vi "DG645_control.vi"() -> ()   [LabVIEW 2016]
uses:
  <vilib>/Utility/xml.llb/Write to XML File(string).vi
  <vilib>/Utility/xml.llb/Read From XML File(string).vi
  <instrlib>/Stanford Research DG645/Stanford Research DG645.lvlib
panel:
  in  "Singl shot":bool
  out "Digital Waveform Graph":digitalwaveform(graph)={"t0"=timestamp(0 s since 1904-01-01), "dt"=4.817138671875e-08, "Y"={"transitions"=[], "data"=array4096x5[20480 elements]}}
  out "Updating":bool
  out "Error":bool
  in  "Reset on update?":bool
  in  "Stop":bool
  in  "Trigger Source":u16(ring)=6 items=["Internal", "External rising edge", "External falling edge", "Single shot internal rising edge", "Single shot external rising edge", "Single shot", "Line"]
  in  "Export to File":bool
  in  "Import From File":bool
  in  "Update Device":bool
  out "error out":errorcluster
  in  "Delays":T1(array[cluster])=[{"Channel"=2, "Reference"=0, "Delay Time"=1e-08}, {"Channel"=3, "Reference"=2, "Delay Time"=1e-05}, {"Channel"=4, "Reference"=2, "Delay Time"=0.000186}, {"Channel"=5, "Reference"=4, "Delay Time"=1e-05}, {"Channel"=6, "Reference"=4, "Delay Time"=3e-07}, {"Channel"=7, "Reference"=6, "Delay Time"=1e-05}, {"Channel"=8, "Reference"=6, "Delay Time"=1e-06}, {"Channel"=9, "Reference"=8, "Delay Time"=1e-05}] {"Delay Time" format="%#_6p"; "Reference" items=["T0"=0, "A"=2, "B"=3, "C"=4, "D"=5, "E"=6, "F"=7, "G"=8, "H"=9]; "Channel" items=["A"=2, "B"=3, "C"=4, "D"=5, "E"=6, "F"=7, "G"=8, "H"=9]}
  in  "Trigger Rate":dbl=50.0
  in  "Outputs":T2(array[cluster])=[{"Output"=0, "Offset"=0.0, "Level"=5.0, "Polarity"=TRUE, "Prescale Factor"=2, "Prescale Phase"=0, "Description"="valve"}, {"Output"=1, "Offset"=0.0, "Level"=5.0, "Polarity"=TRUE, "Prescale Factor"=1, "Prescale Phase"=0, "Description"="flash lamp"}, {"Output"=2, "Offset"=0.0, "Level"=2.7, "Polarity"=TRUE, "Prescale Factor"=1, "Prescale Phase"=0, "Description"="q-switch"}, {"Output"=3, "Offset"=0.0, "Level"=5.0, "Polarity"=TRUE, "Prescale Factor"=1, "Prescale Phase"=0, "Description"="ramp"}, {"Output"=4, "Offset"=0.0, "Level"=5.0, "Polarity"=TRUE, "Prescale Factor"=1, "Prescale Phase"=0, "Description"="scope"}] {"Output" items=["T0", "Output AB", "Output CD", "Output EF", "Output GH"]; "Offset" format="%#_13g"; "Prescale Phase" max=1073741822; "Prescale Factor" min=1 max=1073741823}
  in  "VISA resource name":refnum<visa-resource-name>="DG645_HOGAN"
  # "DG645 control"
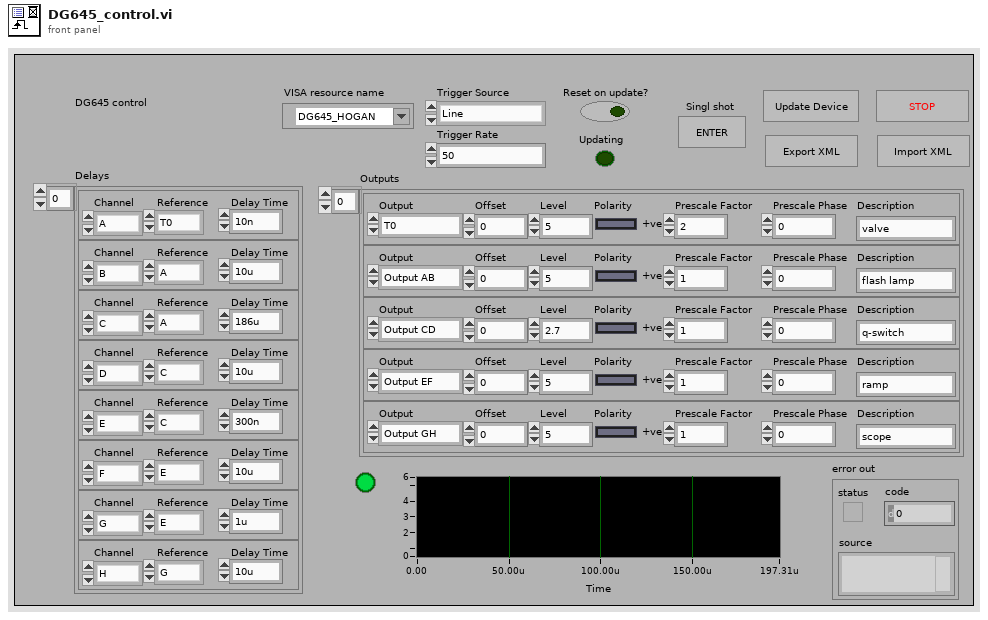
[diagram p1: front panel]
types:
  T1 = cluster{"Channel":u16, "Reference":u16, "Delay Time":dbl}[]
  T2 = cluster{"Output":u16, "Offset":dbl, "Level":dbl, "Polarity":bool, "Prescale Factor":u32, "Prescale Phase":u32, "Description":string}[]
  T3 = cluster{"VISA resource name":refnum<visa-resource-name>, "Trigger Source":u16, "Trigger Rate":dbl, "Delays":cluster{"Channel":u16, "Reference":u16, "Delay Time":dbl}[], "Outputs":cluster{"Output":u16, "Offset":dbl, "Level":dbl, "Polarity":bool, "Prescale Factor":u32, "Prescale Phase":u32, "Description":string}[]}
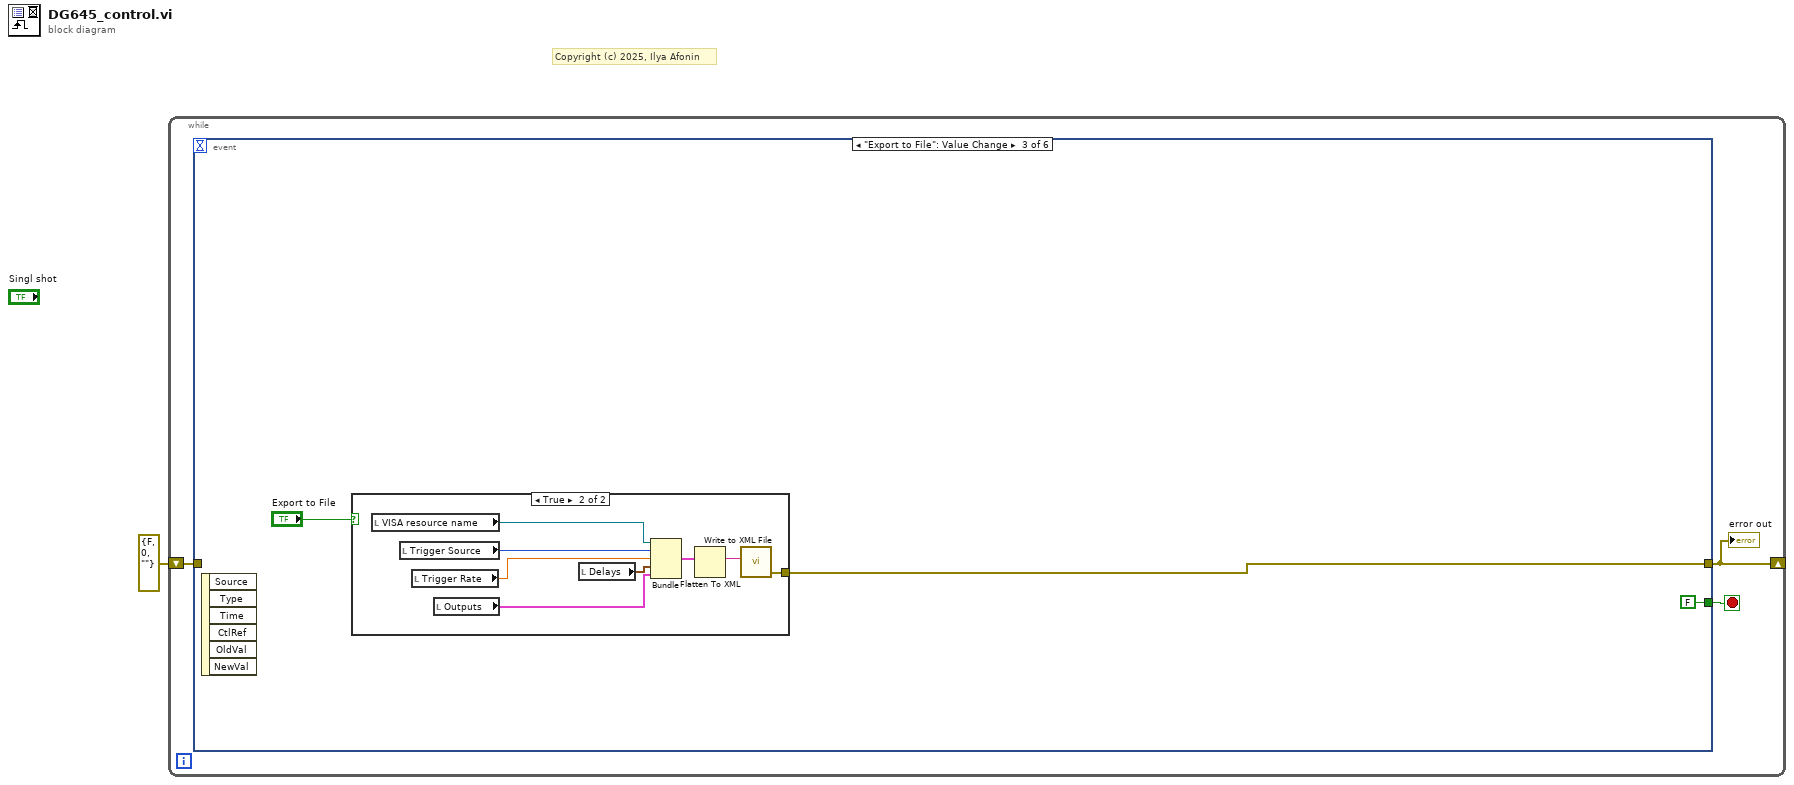
[diagram p0: block diagram]
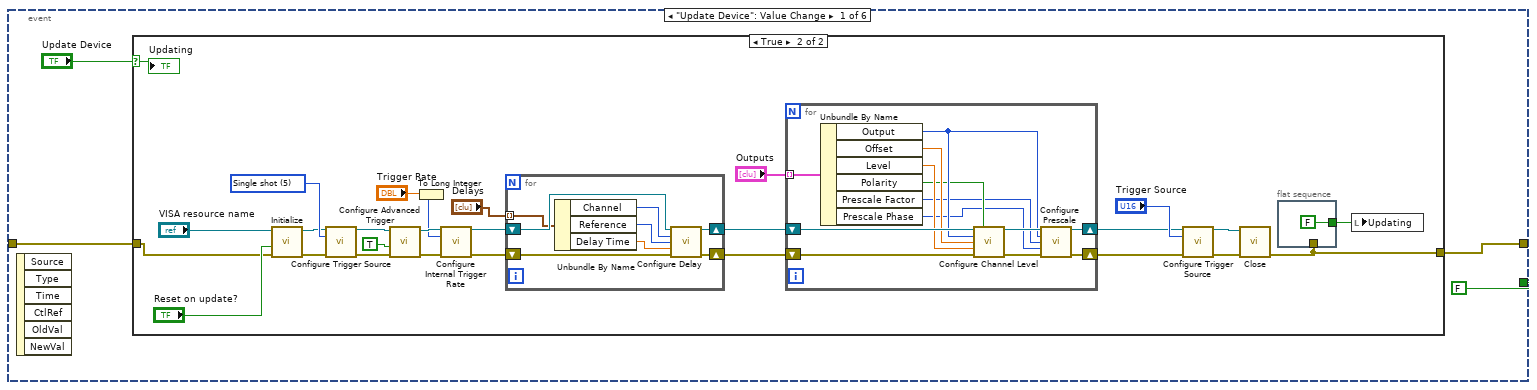
[diagram p2: hidden frame]
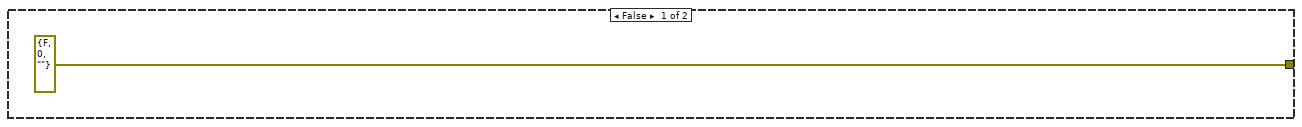
[diagram p3: hidden frame]
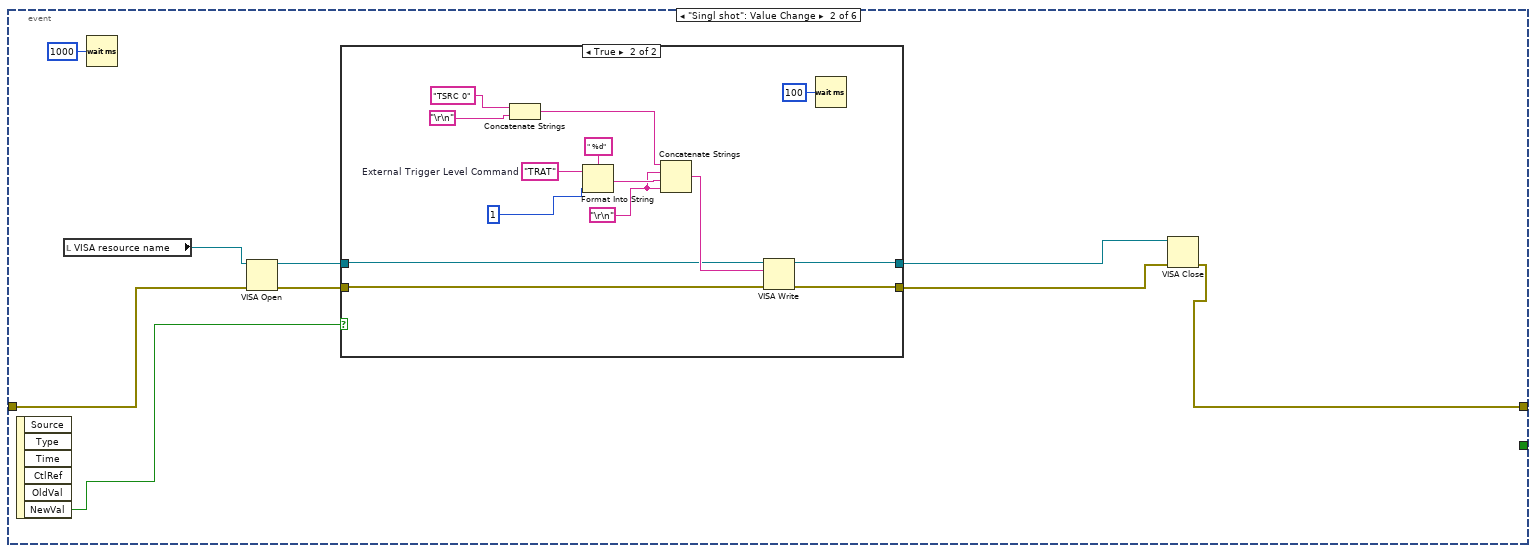
[diagram p4: hidden frame]
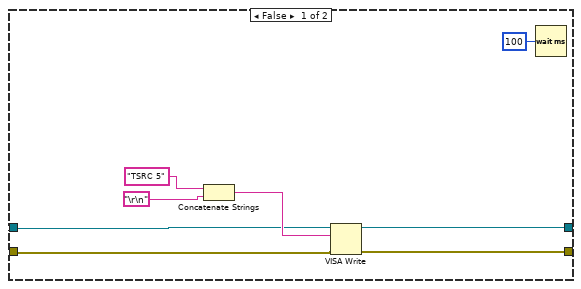
[diagram p5: hidden frame]
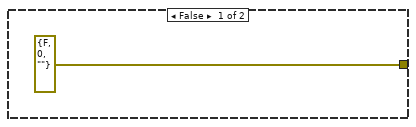
[diagram p6: hidden frame]
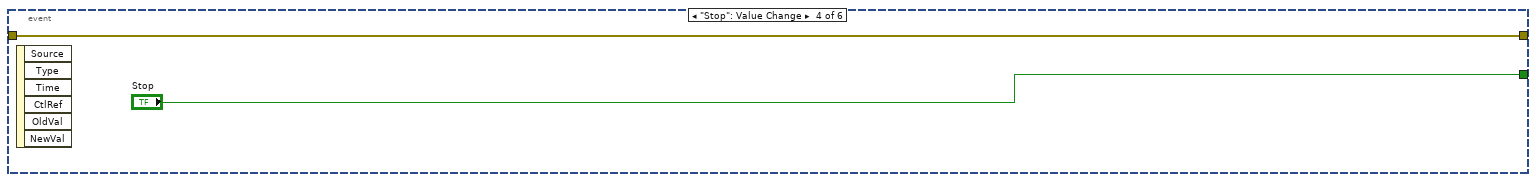
[diagram p7: hidden frame]
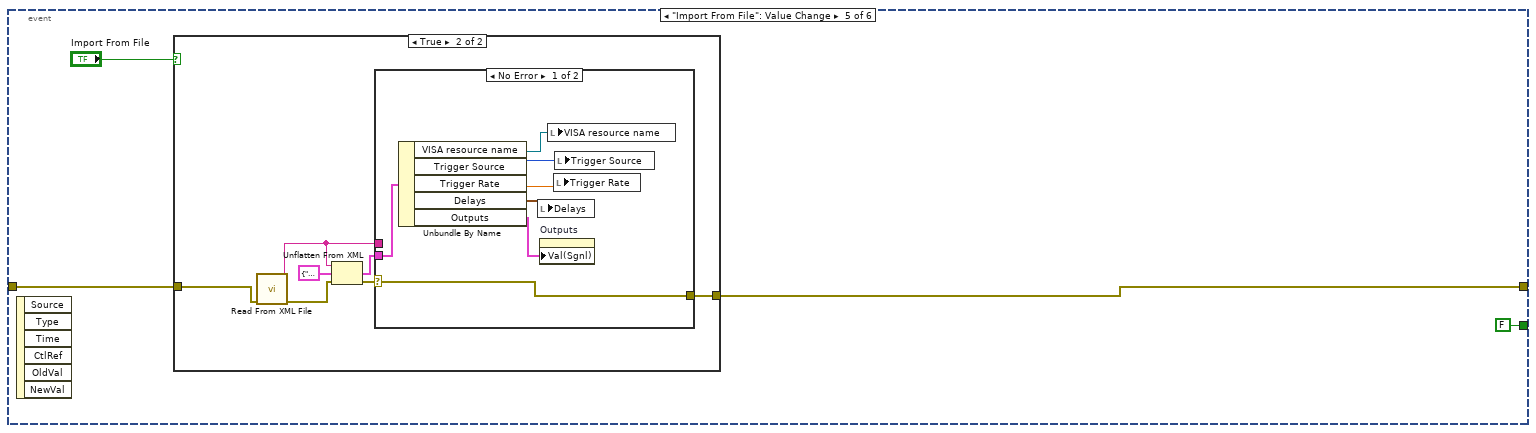
[diagram p8: hidden frame]
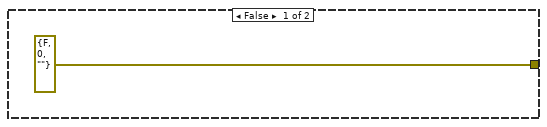
[diagram p9: hidden frame]
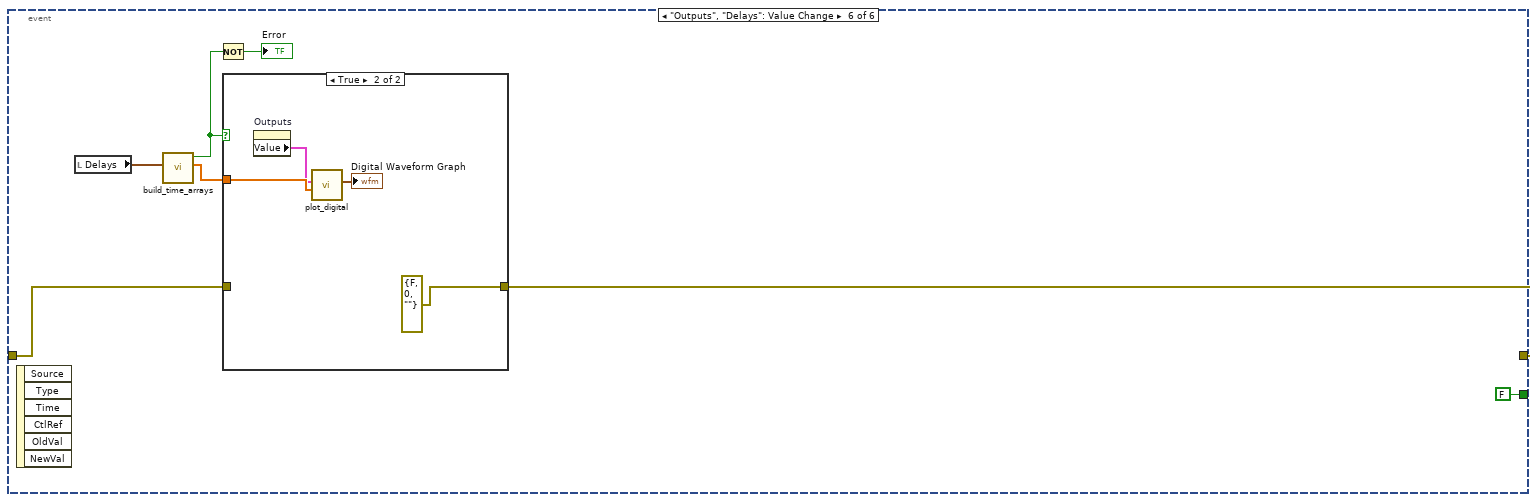
[diagram p11: hidden frame]
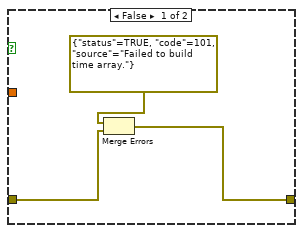
[diagram p12: hidden frame]
diagram:
  # "Copyright (c) 2025, Ilya Afonin"
  n1 = while {
    shift-right: [w3] -> _
    shift-left: errorcluster {"status"=FALSE, "code"=0, "source"=""} ("error out") -> [w2]
    stop <- w4 stop-if-true
    n2 = event shown="[2] \"Export to File\": Value Change" {
      selector: _ -> [_ _ _ _ _ _]
      dyn-events: _ -> [_ _ _ _ _ _]
      timeout: _ -> [_ _ _ _ _ _]
      tunnel: [w8 w63 w92 w102 w107 w129] -> w3
      tunnel: [FALSE ("Stop") _ FALSE ("Stop") "Stop" FALSE ("Stop") FALSE ("Stop")] -> w4
      tunnel: w2 -> [w5 w59 _ w102 w104 w124]
      event "Update Device": Value Change {
        n3 = event-data() -> ()  [unwired: 1 in, 6 out]
        n4 = case shown="True" "Update Device" {
          selector: "Update Device" -> [_ w15]
          tunnel: [errorcluster {"status"=FALSE, "code"=0, "source"=""} ("error out") w14] -> w8
          tunnel: w5 -> [_ w10]
          frame False {
          }
          frame True {
            w23 = u16 5 items=["Internal", "External rising edge", "External falling edge", "Single shot internal rising edge", "Single shot external rising edge", "Single shot", "Line"] ("Trigger Source (5:Single Shot)")
            n5 = call <instrlib>:"Initialize.vi"("error in (no error)"=w10, "Reset (True)"="Reset on update?", "VISA resource name"="VISA resource name") -> ("error out"=w22:errorcluster, "VISA resource name out"=w21:refnum<visa-resource-name>)  [unwired: 7 in]
            n6 = call <instrlib>:"Configure Trigger Source.vi"("VISA resource name"=w21, "Trigger Source (5:Single Shot)"=w23, "error in (no error)"=w22) -> ("VISA resource name out"=w20:refnum<visa-resource-name>, "error out"=w19:errorcluster)  [unwired: 11 in]
            n7 = call <instrlib>:"Configure Advanced Trigger.vi"("error in (no error)"=w19, "Enable Advanced Trigger (False)"=TRUE, "VISA resource name"=w20) -> ("error out"=w29:errorcluster, "VISA resource name out"=w28:refnum<visa-resource-name>)  [unwired: 7 in]
            n8 = To Long Integer(number="Trigger Rate") -> (32bit integer=w11:i32)
            n9 = call <instrlib>:"Configure Internal Trigger Rate.vi"("VISA resource name"=w28, "Internal Trigger Rate (1 MHz)"=w11, "error in (no error)"=w29) -> ("VISA resource name out"=w30:refnum<visa-resource-name>, "error out"=w32:errorcluster)  [unwired: 11 in]
            n10 = for {
              tunnel: "Delays" -> [w43] mode=indexing
              shift-right: [w39] -> w18
              shift-left: w30 -> [w45]
              shift-right: [w38] -> w17
              shift-left: w32 -> [w44]
              n11 = Unbundle By Name(w43) -> ("Channel"=w42:u16, "Reference"=w41:u16, "Delay Time"=w40:dbl)
              n12 = call <instrlib>:"Configure Delay.vi"("VISA resource name"=w45, "Channel to Modify (2:A)"=w42, "Reference Channel (0:T0)"=w41, "Delay Time (0 s)"=w40, "error in (no error)"=w44) -> ("VISA resource name out"=w39:refnum<visa-resource-name>, "error out"=w38:errorcluster)  [unwired: 9 in]
            }
            n13 = for {
              shift-right: [w56] -> w26
              shift-left: w17 -> [w58]
              tunnel: "Outputs" -> [w55] mode=indexing
              shift-right: [w46] -> w16
              shift-left: w18 -> [w57]
              n14 = Unbundle By Name(w55) -> ("Output"=w53:u16, "Offset"=w52:dbl, "Level"=w51:dbl, "Polarity"=w50:bool, "Prescale Factor"=w49:u32, "Prescale Phase"=w48:u32)
              n15 = call <instrlib>:"Configure Channel Level.vi"("VISA resource name"=w57, "Positive Level Polarity (True)"=w50, "Output Channel (0:T0)"=w53, "Level Offset (0 V)"=w52, "Level Amplitude (2.5 V)"=w51, "error in (no error)"=w58) -> ("VISA resource name out"=w54:refnum<visa-resource-name>, "error out"=w47:errorcluster)  [unwired: 8 in]
              n16 = call <instrlib>:"Configure Prescale.vi"("VISA resource name"=w54, "Output Channel (0:T0)"=w53, "Prescale Factor (1)"=w49, "Prescale Phase (0)"=w48, "error in (no error)"=w47) -> ("VISA resource name out"=w46:refnum<visa-resource-name>, "error out"=w56:errorcluster)  [unwired: 9 in]
            }
            n17 = call <instrlib>:"Configure Trigger Source.vi"("VISA resource name"=w16, "Trigger Source (5:Single Shot)"="Trigger Source", "error in (no error)"=w26) -> ("VISA resource name out"=w25:refnum<visa-resource-name>, "error out"=w27:errorcluster)  [unwired: 11 in]
            n18 = call <instrlib>:"Close.vi"("error in (no error)"=w27, "VISA resource name"=w25) -> ("error out"=w14:errorcluster)  [unwired: 9 in]
            n19 = flat-sequence {
              tunnel: w14 -> [_]
              tunnel: [FALSE ("Boolean")] -> w13
              frame #0 {
              }
            }
            n20 = local write "Updating"(w13) -> ()
            "Updating" <- w15
          }
        }
      }
      event "Singl shot": Value Change {
        n21 = event-data() -> ("NewVal"=w67:bool)  [unwired: 1 in, 5 out]
        n22 = local read "VISA resource name"() -> (w60:refnum<visa-resource-name>)
        n23 = Wait (ms)(milliseconds to wait=u32 1000) -> ()  [unwired: 1 out]
        n24 = VISA Open(error in (no error)=w59, VISA resource name=w60) -> (VISA resource name=w61:refnum<visa-resource-name>, error out=w62:errorcluster)  [unwired: 3 in]
        n25 = case shown="True" w67 {
          tunnel: w62 -> [w70 w79]
          tunnel: w61 -> [w71 w80]
          tunnel: [w69 w77] -> w65
          tunnel: [w68 w78] -> w64
          frame False {
            n26 = Concatenate Strings("TSRC 5", "\r\n") -> (w75:string)
            n27 = VISA Write(VISA resource name=w71, write buffer=w75, error in (no error)=w70) -> (VISA resource name out=w69:refnum<visa-resource-name>, error out=w68:errorcluster)  [unwired: 1 out]
            n28 = Wait (ms)(milliseconds to wait=u32 100) -> ()  [unwired: 1 out]
          }
          frame True {
            w81 = "\r\n"
            w89 = "TRAT"  # External Trigger Level Command
            n29 = Concatenate Strings("TSRC 0", "\r\n") -> (w82:string)
            n30 = Format Into String(format string=" %d" ("Source Command"), initial string=w89, 1) -> (resulting string=w87:string)  [unwired: 1 in, 1 out]
            n31 = Concatenate Strings(w82, w81, w87, w81) -> (w86:string)
            n32 = VISA Write(VISA resource name=w80, write buffer=w86, error in (no error)=w79) -> (VISA resource name out=w77:refnum<visa-resource-name>, error out=w78:errorcluster)  [unwired: 1 out]
            n33 = Wait (ms)(milliseconds to wait=u32 100) -> ()  [unwired: 1 out]
          }
        }
        n34 = VISA Close(VISA resource name=w65, error in (no error)=w64) -> (error out=w63:errorcluster)
      }
      event "Export to File": Value Change {
        n35 = event-data() -> ()  [unwired: 1 in, 6 out]
        n36 = case shown="True" "Export to File" {
          tunnel: [errorcluster {"status"=FALSE, "code"=0, "source"=""} ("error out") w94] -> w92
          frame False {
          }
          frame True {
            n37 = local read "VISA resource name"() -> (w101:refnum<visa-resource-name>)
            n38 = local read "Trigger Source"() -> (w100:u16)
            n39 = local read "Trigger Rate"() -> (w99:dbl)
            n40 = local read "Outputs"() -> (w97:T2)
            n41 = local read "Delays"() -> (w98:T1)
            n42 = Bundle("VISA resource name"=w101, "Trigger Source"=w100, "Trigger Rate"=w99, "Delays"=w98, "Outputs"=w97) -> (w96:T3)  [unwired: 1 in]
            n43 = Flatten To XML(anything=w96) -> (xml string=w95:string)
            n44 = call-poly <vilib>:"Write to XML File.vi"("XML Input"=w95) -> ("error out"=w94:errorcluster)  [unwired: 8 in, 2 out]
          }
        }
      }
      event "Stop": Value Change {
        n45 = event-data() -> ()  [unwired: 1 in, 6 out]
      }
      event "Import From File": Value Change {
        n46 = event-data() -> ()  [unwired: 1 in, 6 out]
        n47 = case shown="True" "Import From File" {
          tunnel: [errorcluster {"status"=FALSE, "code"=0, "source"=""} ("error out") w112] -> w107
          tunnel: w104 -> [_ w109]
          frame False {
          }
          frame True {
            n48 = call-poly <vilib>:"Read From XML File.vi"("error in (no error)"=w109) -> ("error out"=w111:errorcluster, "XML Elements"=w110:string)  [unwired: 8 in, 1 out]
            n49 = Unflatten From XML(xml string=w110, type=T3 {"VISA resource name"="", "Trigger Source"=0, "Trigger Rate"=0.0, "Delays"=[], "Outputs"=[]} ("output cluster"), error in (no error)=w111) -> (value=w114:T3, error out=w113:errorcluster)
            n50 = case shown="No Error" w113 {
              selector: w113 -> [w121 w123]
              tunnel: w114 -> [w122 _]
              tunnel: [w121 w123] -> w112
              tunnel: w110 -> [_ _]
              frame No Error {
                n51 = Unbundle By Name(w122) -> ("VISA resource name"=w120:refnum<visa-resource-name>, "Trigger Source"=w119:u16, "Trigger Rate"=w118:dbl, "Delays"=w117:T1, "Outputs"=w116:T2)
                n52 = local write "Delays"(w117) -> ()
                n53 = property on="Outputs" class="Arr (strict)"("Val(Sgnl)"=w116) -> ()  [unwired: 2 in, 2 out]
                n54 = local write "VISA resource name"(w120) -> ()
                n55 = local write "Trigger Rate"(w118) -> ()
                n56 = local write "Trigger Source"(w119) -> ()
              }
              frame Error {
              }
            }
          }
        }
      }
      event "Outputs", "Delays": Value Change {
        n57 = event-data() -> ()  [unwired: 1 in, 6 out]
        n58 = local read "Delays"() -> (w128:T1)
        n59 = call "build_time_arrays.vi"("Delays"=w128) -> ("Array"=w127:dbl[], "ok"=w126:bool)  [unwired: 9 in]
        n60 = Not(x=w126) -> (.not. x?=→"Error":bool)
        n61 = case shown="True" w126 {
          tunnel: w127 -> [_ w136]
          tunnel: [w132 errorcluster {"status"=FALSE, "code"=0, "source"=""} ("error out")] -> w129
          tunnel: w124 -> [w133 _]
          frame False {
            n62 = Merge Errors(errorcluster {"status"=TRUE, "code"=101, "source"="Failed to build time array."} ("error out"), w133) -> (w132:errorcluster)
          }
          frame True {
            n63 = property on="Outputs" class="Arr (strict)"() -> ("Value"=w135:T2)  [unwired: 2 in, 2 out]
            n64 = call "plot_digital.vi"("array"=w136, "Outputs"=w135) -> ("Digital Waveform Graph"=→"Digital Waveform Graph":digitalwaveform)  [unwired: 9 in]
          }
        }
      }
    }
    "error out" <- w3
  }
